vi "Reset Saftey Relay.vi"(4 "error in":errorcluster) -> (0 "error out":errorcluster, 2 "System Reset pressed?":bool)   [LabVIEW 2015]
uses:
  <vilib>/DAQmx/read.llb/DAQmx Read (Digital Bool 1Line 1Point).vi
  <vilib>/DAQmx/miscellaneous.llb/DAQmx Fill In Error Info.vi
  <vilib>/DAQmx/write.llb/DAQmx Write (Digital Bool 1Line 1Point).vi
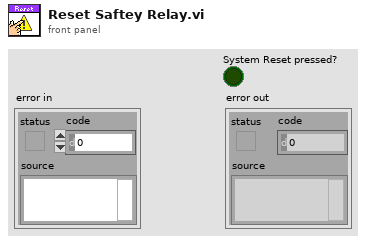
[diagram p1: front panel]
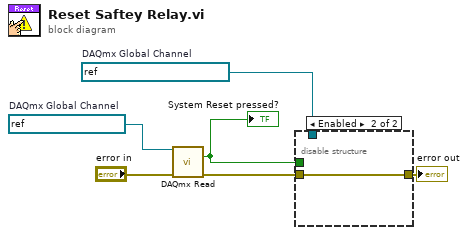
[diagram p0: block diagram]
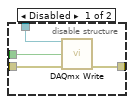
[diagram p2: hidden frame]
diagram:
  w4 = refnum<k21> "DO0 Reset Safety Relay"  # DAQmx Global Channel
  w5 = refnum<k21> "DI4 System Reset"  # DAQmx Global Channel
  n1 = call-poly <vilib>:"DAQmx Read.vi"("task/channels in"=w5, "error in"="error in") -> ("data"=w6:bool, "error out"=w3:errorcluster)  [unwired: 11 in, 1 out]
  "System Reset pressed?" <- w6
  n2 = disable-structure shown="Enabled" {
    disable-tunnel: w6 -> [w10 _]
    disable-tunnel: w4 -> [w9 _]
    disable-tunnel: w3 -> [w8 w11]
    disable-tunnel: [w7 w11] -> w1
    frame Disabled {
      n3 = call-poly <vilib>:"DAQmx Write.vi"("task/channels in"=w9, "data"=w10, "error in"=w8) -> ("error out"=w7:errorcluster)  [unwired: 10 in, 2 out]
    }
    frame Enabled {
    }
  }
  "error out" <- w1
